vi "Set Remote Lockout.vi"(0 "VISA resource name":refnum<visa-resource-name>, 5 "System Mode (0: Local)":i32(ring) items=["Local", "Remote", "Remote with Lock"], 11 "error in (no error)":errorcluster) -> (4 "VISA resource name out":refnum<visa-resource-name>, 15 "error out":errorcluster)   [LabVIEW 2012, in "NH Research Regenerative Test Series.lvlib"]
doc: "This will place the module in either local, remote, or remote with lock mode during SCPI operation."
uses:
  <instrlib>/NH Research Regenerative Test Series/NH Research Regenerative Test Series.lvlib
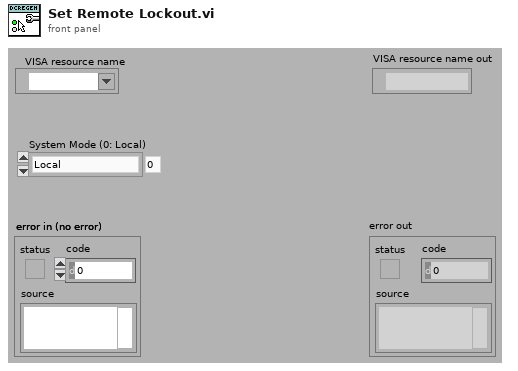
[diagram p1: front panel]
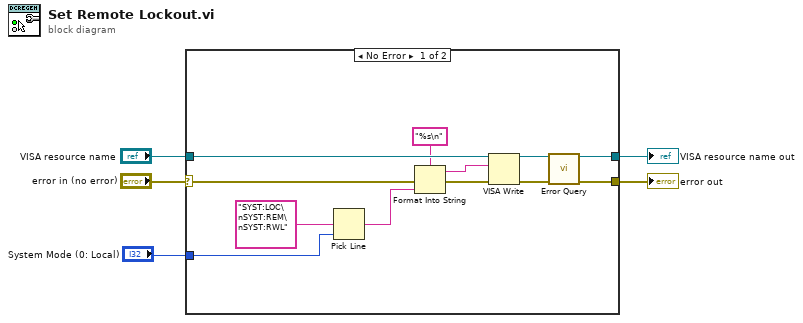
[diagram p0: block diagram]
diagram:
  n1 = case shown="No Error" "error in (no error)" {
    selector: "error in (no error)" -> [w12 w19]
    tunnel: "VISA resource name" -> [w17 w18]
    tunnel: [w16 w18] -> w4
    tunnel: [w15 w19] -> w3
    tunnel: "System Mode (0: Local)" -> [w7 _]
    frame No Error {
      n2 = Pick Line(multi-line string="SYST:LOC\nSYST:REM\nSYST:RWL", line index=w7) -> (output string=w6:string)  [unwired: 1 in]
      n3 = Format Into String(format string="%s\n", error in=w12, w6) -> (resulting string=w9:string, error out=w10:errorcluster)  [unwired: 1 in]
      n4 = VISA Write(VISA resource name=w17, write buffer=w9, error in (no error)=w10) -> (VISA resource name out=w14:refnum<visa-resource-name>, error out=w13:errorcluster)  [unwired: 1 out]
      n5 = call <instrlib>:"Error Query.vi"("VISA resource name"=w14, "error in (no error)"=w13) -> ("VISA resource name out"=w16:refnum<visa-resource-name>, "error out"=w15:errorcluster)  [unwired: 10 in, 2 out]
    }
    frame Error {
    }
  }
  "error out" <- w3
  "VISA resource name out" <- w4
